vi "KE622x -- 2182 -A Clear Output Buf.vi"(0 "622x Resource In":refnum<visa-resource-name>, 1 "Check For SCPI Errors? (T)":bool=TRUE, 7 "Num Reads (1)":i32=1 min=1 max=100, 9 "Max Num Bytes To Read (256)":u32=256, 11 "error in (no error)":errorcluster) -> (4 "622x Resource Out (dupl)":refnum<visa-resource-name>, 8 "Responses":string[](array[string]), 15 "error out":errorcluster)   [LabVIEW 2019, in "Keithley 622x.lvlib"]
uses:
  Keithley 622x.lvlib
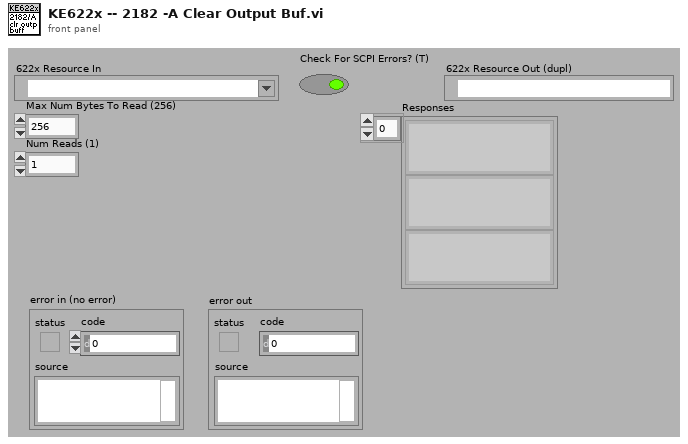
[diagram p1: front panel]
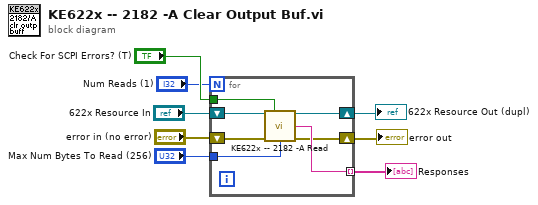
[diagram p0: block diagram]
diagram:
  n1 = for {
    N: "Num Reads (1)" -> [_]
    tunnel: "Check For SCPI Errors? (T)" -> [w15]
    shift-right: [w10] -> w2
    shift-left: "622x Resource In" -> [w14]
    shift-right: [w11] -> w1
    shift-left: "error in (no error)" -> [w13]
    tunnel: [w12] -> w4 mode=indexing
    tunnel: "Max Num Bytes To Read (256)" -> [w9]
    n2 = call "KE622x -- 2182 -A Read.vi"("622x Resource In"=w14, "Check For SCPI Errors? (T)"=w15, "error in (no error)"=w13, "Max Num Bytes To Read (256)"=w9) -> ("622x Resource Out (dupl)"=w10:refnum<visa-resource-name>, "2182-A Reponse String"=w12:string, "error out"=w11:errorcluster)  [unwired: 9 in]
  }
  "622x Resource Out (dupl)" <- w2
  "error out" <- w1
  "Responses" <- w4
